vi "write_log_spike_data_1.vi"(8 "error in (no error)":errorcluster, 10 "Cluster 2":T1, 11 "Log File in":refnum<k34>) -> (0 "error out":errorcluster, 3 "Log File out":refnum<k34>)   [LabVIEW 2017]
uses:
  Control 2.ctl
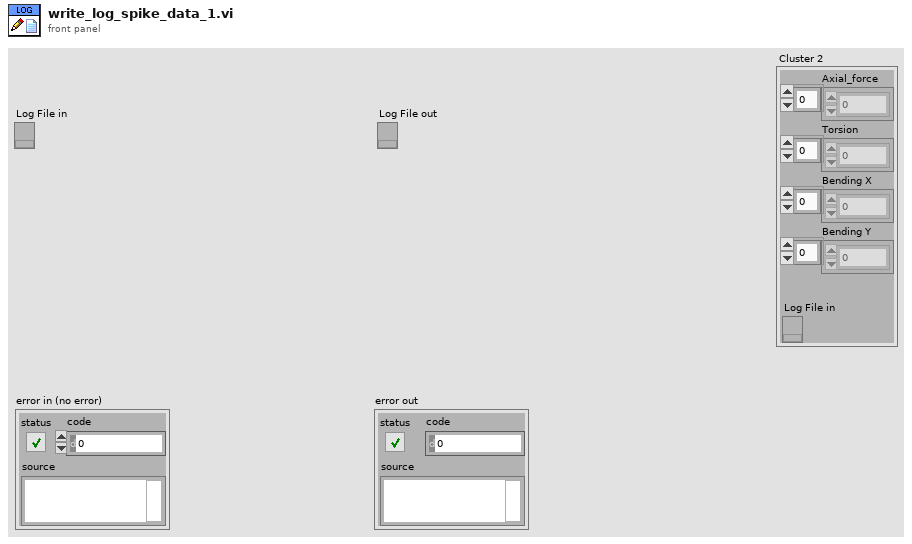
[diagram p1: front panel]
types:
  T1 = typedef "Control 2.ctl" = cluster{"Axial_force":i16[], "Torsion":i16[], "Bending X":i16[], "Bending Y":i16[], "Log File in":refnum<k34>}
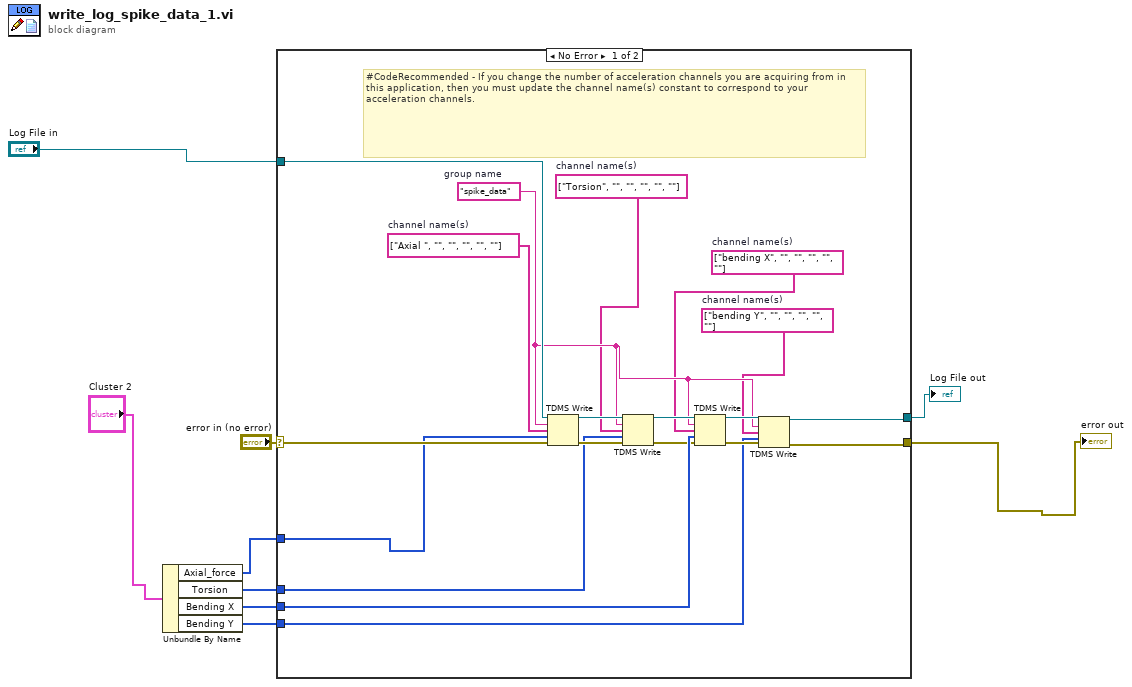
[diagram p0: block diagram]
diagram:
  n1 = Unbundle By Name("Cluster 2") -> ("Axial_force"=w5:i16[], "Torsion"=w4:i16[], "Bending X"=w3:i16[], "Bending Y"=w2:i16[])
  n2 = case shown="No Error" "error in (no error)" {
    selector: "error in (no error)" -> [w26 w29]
    tunnel: "Log File in" -> [w27 w30]
    tunnel: [w21 w30] -> w8
    tunnel: [w18 w29] -> w6
    tunnel: w5 -> [w25 _]
    tunnel: w4 -> [w13 _]
    tunnel: w3 -> [w12 _]
    tunnel: w2 -> [w11 _]
    frame No Error {
      w14 = string[] ["bending Y", "", "", "", "", ""]  # channel name(s)
      w15 = string[] ["bending X", "", "", "", "", ""]  # channel name(s)
      w16 = string[] ["Torsion", "", "", "", "", ""]  # channel name(s)
      w28 = string[] ["Axial ", "", "", "", "", ""]  # channel name(s)
      w17 = "spike_data"  # group name
      # "#CodeRecommended - If you change the number of acceleration channels you are acquiring from in this application, then you must update the channel name(s) constant to correspond to your acceleration channels."
      n3 = TDMS Write(0:w27, 5:w17, 7:w28, 9:w25, 11:w26) -> (4:w24:refnum<k34>, 15:w20:errorcluster)  [unwired: 1 in, 2 out]
      n4 = TDMS Write(0:w24, 5:w17, 7:w16, 9:w13, 11:w20) -> (4:w23:refnum<k34>, 15:w10:errorcluster)  [unwired: 1 in, 2 out]
      n5 = TDMS Write(0:w23, 5:w17, 7:w15, 9:w12, 11:w10) -> (4:w22:refnum<k34>, 15:w19:errorcluster)  [unwired: 1 in, 2 out]
      n6 = TDMS Write(0:w22, 5:w17, 7:w14, 9:w11, 11:w19) -> (4:w21:refnum<k34>, 15:w18:errorcluster)  [unwired: 1 in, 2 out]
    }
    frame Error {
    }
  }
  "Log File out" <- w8
  "error out" <- w6
